vi "Read ActiveEffect.vi"(8 "error in (no error)":errorcluster, 11 "Grape in":refnum<class "Grape.lvclass">) -> (0 "error out":errorcluster, 2 "ActiveEffect":bool, 3 "Grape out":refnum<class "Grape.lvclass">)   [LabVIEW 2021, in "Grape.lvclass"]
uses:
  Grape.lvclass
  Grape.lvclass/Grape.ctl
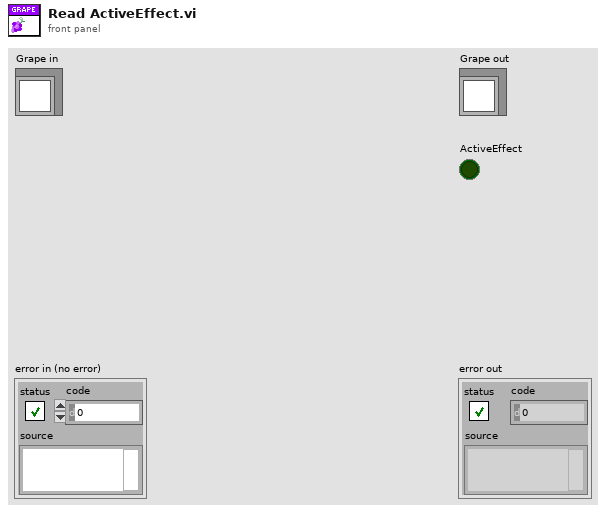
[diagram p1: front panel]
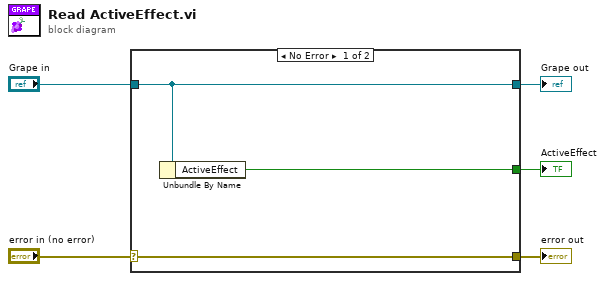
[diagram p0: block diagram]
diagram:
  n1 = case shown="No Error" "error in (no error)" {
    selector: "error in (no error)" -> [w8 w9]
    tunnel: [w8 w9] -> w4
    tunnel: [w7 w10] -> w2
    tunnel: "Grape in" -> [w7 w10]
    tunnel: [w6 _] -> w1
    frame No Error {
      n2 = Unbundle By Name(w7) -> ("ActiveEffect"=w6:bool)
    }
    frame Error {
    }
  }
  "error out" <- w4
  "Grape out" <- w2
  "ActiveEffect" <- w1
